vi "Maxi Gauge - Example.vi"(8 "error in (no error)":errorcluster caption="Fehler (Eingang, kein Fehler)", 10 "Sensor Nr.:":i32(ring) items=["sensor 1", "sensor 2", "sensor 3", "sensor 4", "sensor 5", "sensor 6"], 11 "input refnum":refnum<visa-resource-name> caption="Eingang (Referenz)") -> (0 "error out":errorcluster, 1 "Pressure":dbl format="%.3e", 2 "Status":i32(ring) items=["data OK", "underrange", "overrange", "sensor error", "sensor off", "no sensor", "ID error"])   [LabVIEW 2012, in "Maxi Gauge.lvlib"]
uses:
  Maxi Gauge.lvlib
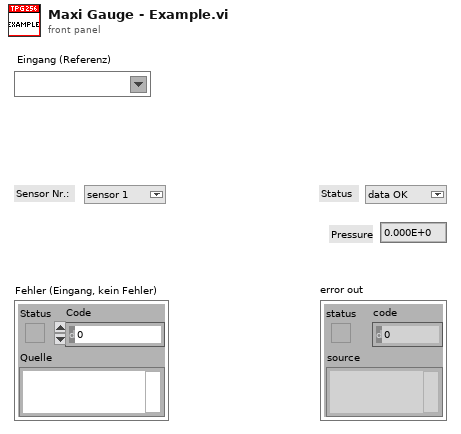
[diagram p1: front panel]
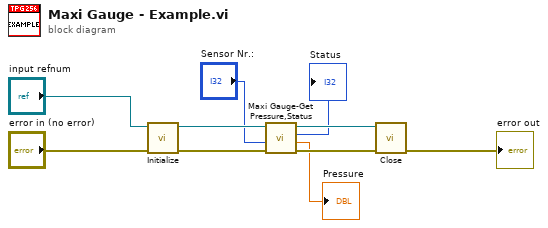
[diagram p0: block diagram]
diagram:
  n1 = call "Initialize.vi"("error in (no error)"="error in (no error)", "input refnum"="input refnum") -> ("error out"=w5:errorcluster, "VISA resource out"=w7:refnum<visa-resource-name>)  [unwired: 8 in]
  n2 = call "Maxi Gauge-Get Pressure,Status.vi"("Fehler (Eingang, kein Fehler)"=w5, "Sensor Nr.:"="Sensor Nr.:", "VISA-Ressource in"=w7) -> ("Fehler (Ausgang)"=w4:errorcluster, "Pressure"=→"Pressure":dbl, "Status"=→"Status":i32, "VISA-Ressource out"=w6:refnum<visa-resource-name>)  [unwired: 5 in]
  n3 = call "Close.vi"("error in (no error)"=w4, "VISA resource name"=w6) -> ("error out"=→"error out":errorcluster)  [unwired: 9 in]
